vi "读取流量传感器(子VI).vi"() -> (0 "结果":bool, 1 "R(Gas)mv":string, 2 "F(Flow)ml/min":string, 3 "P（eq)mv":string, 4 "T(cool)℃":string)   [LabVIEW 2016]
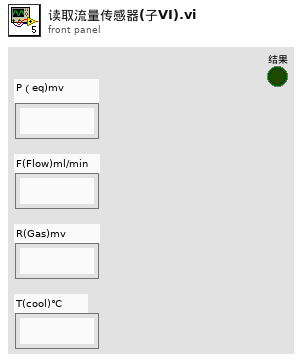
[diagram p1: front panel]
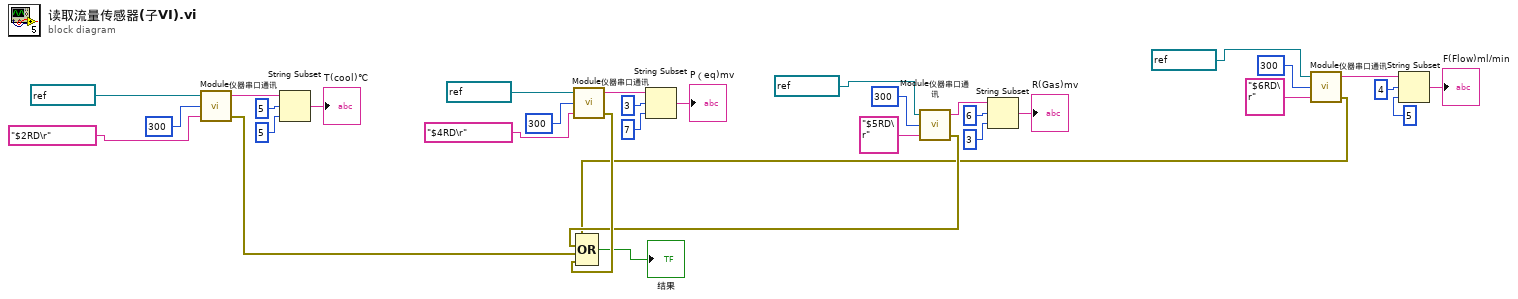
[diagram p0: block diagram]
diagram:
  n1 = call "Module仪器串口通讯.vi"("输入指令"="$2RD\r", "baud rate"=u32 300 ("baud rate (9600)"), "VISA resource name"=refnum<visa-resource-name> "COM3") -> ("错误输出"=w5:errorcluster, "子字符串;substring"=w12:string)  [unwired: 1 out]
  n2 = String Subset(string=w12, offset (0)=5 ("偏移量(0)"), length (rest)=5 ("长度（剩余）")) -> (substring=→"T(cool)℃":string)
  n3 = call "Module仪器串口通讯.vi"("输入指令"="$4RD\r", "baud rate"=u32 300 ("baud rate (9600)"), "VISA resource name"=refnum<visa-resource-name> "COM3") -> ("错误输出"=w4:errorcluster, "子字符串;substring"=w19:string)  [unwired: 1 out]
  n4 = String Subset(string=w19, offset (0)=3 ("偏移量(0)"), length (rest)=7 ("长度（剩余）")) -> (substring=→"P（eq)mv":string)
  n5 = call "Module仪器串口通讯.vi"("输入指令"="$5RD\r", "baud rate"=u32 300 ("baud rate (9600)"), "VISA resource name"=refnum<visa-resource-name> "COM3") -> ("错误输出"=w3:errorcluster, "子字符串;substring"=w26:string)  [unwired: 1 out]
  n6 = String Subset(string=w26, offset (0)=6 ("偏移量(0)"), length (rest)=3 ("长度（剩余）")) -> (substring=→"R(Gas)mv":string)
  n7 = call "Module仪器串口通讯.vi"("输入指令"="$6RD\r", "baud rate"=u32 300 ("baud rate (9600)"), "VISA resource name"=refnum<visa-resource-name> "COM3") -> ("错误输出"=w2:errorcluster, "子字符串;substring"=w33:string)  [unwired: 1 out]
  n8 = Compound Arithmetic op=OR ("复合运算")(w2, w3, w5, w4) -> (→"结果":bool)
  n9 = String Subset(string=w33, offset (0)=4 ("偏移量(0)"), length (rest)=5 ("长度（剩余）")) -> (substring=→"F(Flow)ml/min":string)
